vi "GEA2 Extract 2017 Washer.vi"(8 "Error In":errorcluster, 9 "ERD Number":u16 format="%x", 10 "Data":string, 11 "ERD Headers":string[](array[string])) -> (0 "Error Out":errorcluster, 3 "Array":string[][](array[string]))   [LabVIEW 2016, in "GEA2_Toolkit.lvlib"]
uses:
  library/GEA2_Toolkit.lvlib
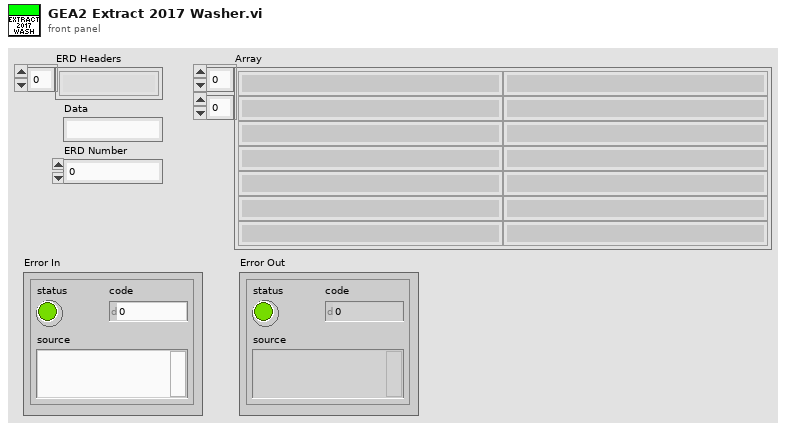
[diagram p1: front panel]
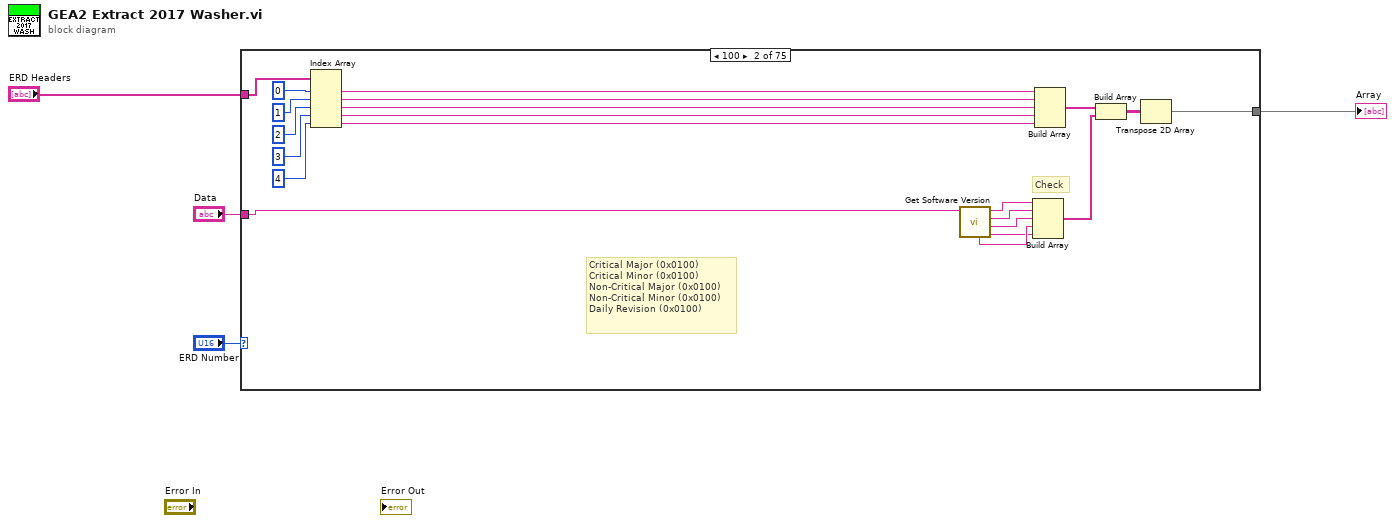
[diagram p0: block diagram]
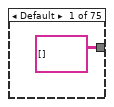
[diagram p2: hidden frame]
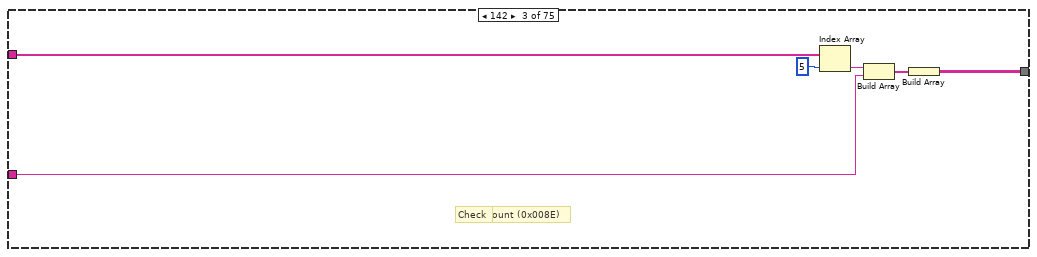
[diagram p3: hidden frame]
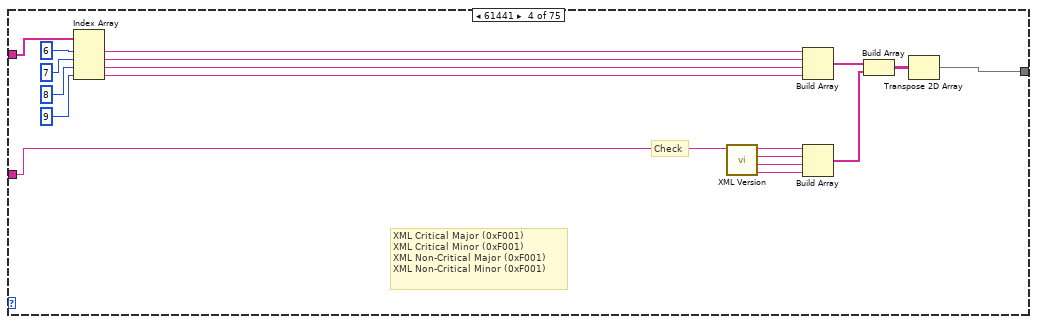
[diagram p4: hidden frame]
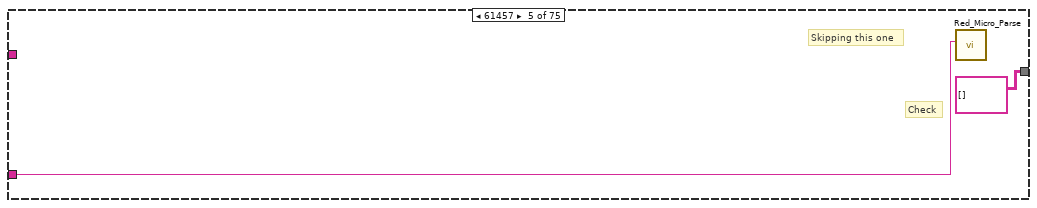
[diagram p5: hidden frame]
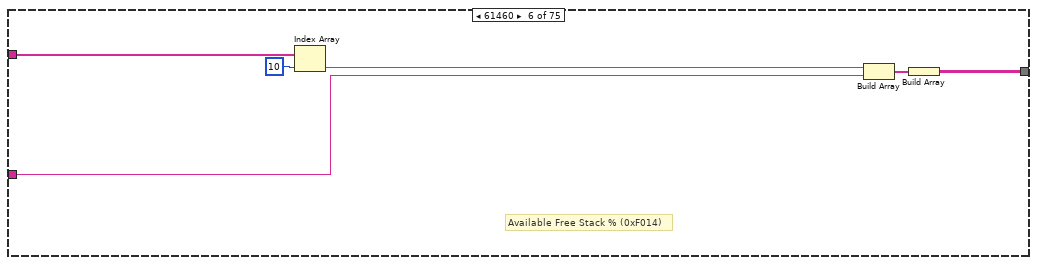
[diagram p6: hidden frame]
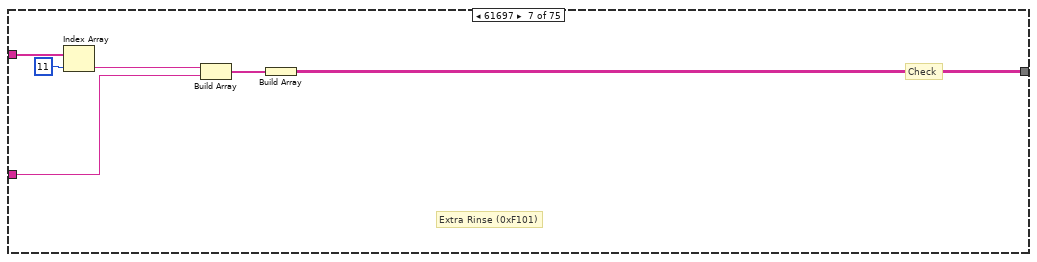
[diagram p7: hidden frame]
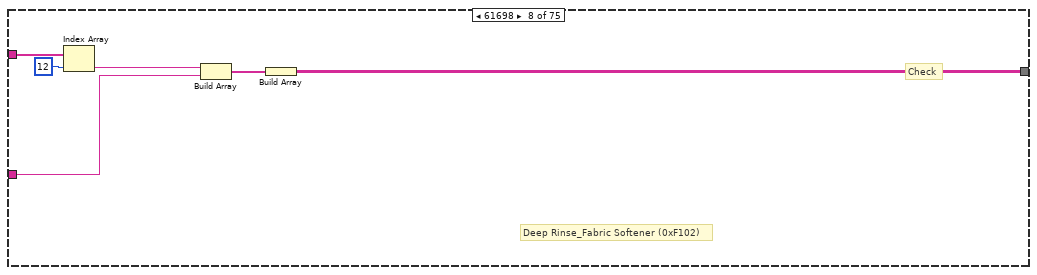
[diagram p8: hidden frame]
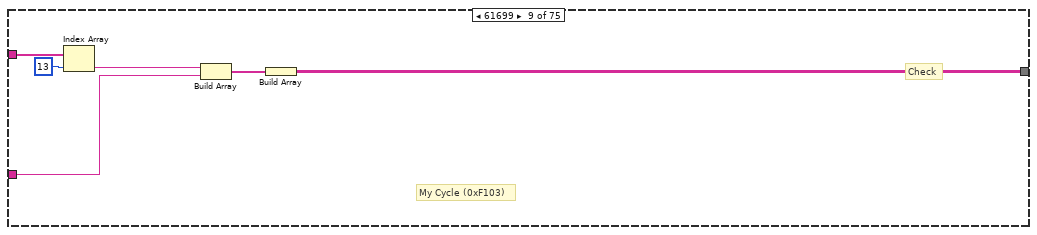
[diagram p9: hidden frame]
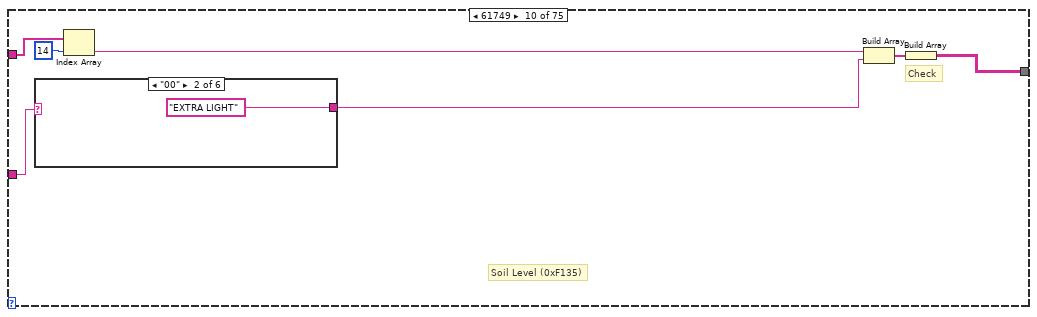
[diagram p10: hidden frame]
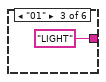
[diagram p12: hidden frame]
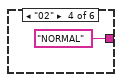
[diagram p13: hidden frame]
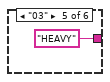
[diagram p14: hidden frame]
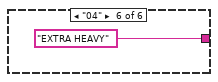
[diagram p15: hidden frame]
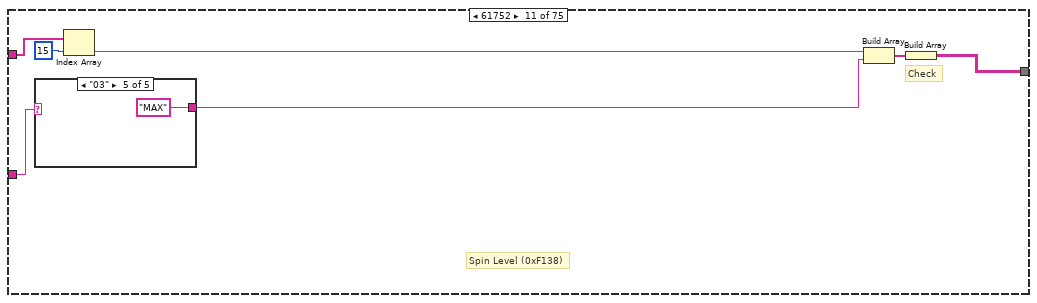
[diagram p16: hidden frame]
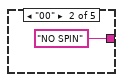
[diagram p18: hidden frame]
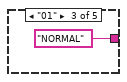
[diagram p19: hidden frame]
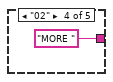
[diagram p20: hidden frame]
diagram:
  n1 = case shown="100" "ERD Number" {
    tunnel: "Data" -> [_ w26 w27 w50 w52 w53 w59 w65 w71 w83 w96 w108 w122 w136 w149 w157 w175 w181 w188 w199 w206 w212 w219 w230 w241 w252 w268 w282 w313 w323 w336 w342 w349 w364 w374 w384 w393 w409 w419 w424 w434 w444 w454 w464 w486 w500 w501 w508 w518 w527 w534 w540 w546 w553 w566 w588 w610 w625 w631 w638 w654 w671 w680 w686 w692 w709 w730 w737 w743 w749 w761 w762 w769 w775 w791]
    tunnel: [string[][] [] w6 w28 w33 string[][] [] w54 w60 w66 w72 w77 w90 w102 w116 w130 w143 w151 w176 w182 w187 w193 w207 w213 w224 w231 w242 w253 w262 w284 w288 w316 w330 w343 w350 w358 w368 w378 w394 w403 w413 w425 w435 w445 w455 w465 w473 w487 w503 w511 w519 w528 w535 w541 w547 w554 w559 w581 w603 w626 w632 w639 w647 w665 w681 w687 w693 w698 w724 w738 w744 w750 w756 w763 w770 w776 w781] -> w4
    tunnel: "ERD Headers" -> [_ w8 w32 w49 _ w58 w64 w67 w73 w79 w92 w103 w118 w132 w145 w153 w177 w183 w189 w195 w208 w214 w225 w232 w243 w255 w264 w285 w293 w319 w331 w344 w353 w359 w370 w380 w398 w404 w415 w428 w438 w446 w456 w468 w478 w492 w502 w512 w522 w530 w536 w542 w548 w555 w562 w582 w606 w627 w633 w640 w648 w667 w682 w688 w694 w701 w726 w739 w745 w751 w757 w764 w771 w777 w782]
    frame Default {
    }
    frame 256 {
      # "Critical Major (0x0100)\nCritical Minor (0x0100)\nNon-Critical Major (0x0100)\nNon-Critical Minor (0x0100)\nDaily Revision (0x0100)"
      # "Check"
      n2 = Index Array(array=w8, index #1=0 ("index"), index #2=1 ("index"), index #3=2 ("index"), index #4=3 ("index"), index #5=4 ("index")) -> (element #1=w20:string, element #2=w19:string, element #3=w18:string, element #4=w17:string, element #5=w16:string)
      n3 = call "Get Software Version.vi"("Data"=w26) -> ("Daily Revision"=w11:string, "Non-Critical Major"=w13:string, "Critical Minor"=w14:string, "Critical Major"=w15:string, "Non-Critical Minor"=w12:string)  [unwired: 6 in]
      n4 = Build Array(w15, w14, w13, w12, w11) -> (w9:string[])
      n5 = Build Array(w20, w19, w18, w17, w16) -> (w10:string[])
      n6 = Build Array(w10, w9) -> (w7:string[][])
      n7 = Transpose 2D Array(2D array=w7) -> (transposed array=w6:string[][])
    }
    frame 142 {
      # "Cycle Count (0x008E)"
      # "Check"
      n8 = Index Array(array=w32, index=5) -> (element=w30:string)
      n9 = Build Array(w30, w27) -> (w29:string[])
      n10 = Build Array(w29) -> (w28:string[][])
    }
    frame 61441 {
      # "XML Critical Major (0xF001)\nXML Critical Minor (0xF001)\nXML Non-Critical Major (0xF001)\nXML Non-Critical Minor (0xF001)"
      # "Check"
      n11 = Index Array(array=w49, index #1=6 ("index"), index #2=7 ("index"), index #3=8 ("index"), index #4=9 ("index")) -> (element #1=w44:string, element #2=w43:string, element #3=w42:string, element #4=w41:string)
      n12 = call "XML Version.vi"("Data"=w50) -> ("XML Non-Critical Minor"=w37:string, "XML Non-Critical Major"=w38:string, "XML Critical Minor"=w39:string, "XML Critical Major"=w40:string)  [unwired: 7 in]
      n13 = Build Array(w44, w43, w42, w41) -> (w36:string[])
      n14 = Build Array(w40, w39, w38, w37) -> (w35:string[])
      n15 = Build Array(w36, w35) -> (w34:string[][])
      n16 = Transpose 2D Array(2D array=w34) -> (transposed array=w33:string[][])
    }
    frame 61457 {
      # "Skipping this one"
      # "Check"
      n17 = call "Red_Micro_Parse.vi"("Data"=w52) -> ()  [unwired: 10 in, 1 out]
    }
    frame 61460 {
      # "Available Free Stack % (0xF014)"
      n18 = Index Array(array=w58, index=10) -> (element=w56:string)
      n19 = Build Array(w56, w53) -> (w55:string[])
      n20 = Build Array(w55) -> (w54:string[][])
    }
    frame 61697 {
      # "Extra Rinse (0xF101)"
      # "Check"
      n21 = Index Array(array=w64, index=11) -> (element=w62:string)
      n22 = Build Array(w62, w59) -> (w61:string[])
      n23 = Build Array(w61) -> (w60:string[][])
    }
    frame 61698 {
      # "Deep Rinse_Fabric Softener (0xF102)"
      # "Check"
      n24 = Index Array(array=w67, index=12) -> (element=w69:string)
      n25 = Build Array(w69, w65) -> (w68:string[])
      n26 = Build Array(w68) -> (w66:string[][])
    }
    frame 61699 {
      # "My Cycle (0xF103)"
      # "Check"
      n27 = Index Array(array=w73, index=13) -> (element=w75:string)
      n28 = Build Array(w75, w71) -> (w74:string[])
      n29 = Build Array(w74) -> (w72:string[][])
    }
    frame 61749 {
      # "Soil Level (0xF135)"
      # "Check"
      n30 = case shown="\"00\"" w83 {
        selector: w83 -> [w84 _ _ _ _ _]
        tunnel: [w84 "EXTRA LIGHT" "LIGHT" "NORMAL" "HEAVY" "EXTRA HEAVY"] -> w78
        frame Default {
        }
        frame "00" {
        }
        frame "01" {
        }
        frame "02" {
        }
        frame "03" {
        }
        frame "04" {
        }
      }
      n31 = Index Array(array=w79, index=14) -> (element=w81:string)
      n32 = Build Array(w81, w78) -> (w80:string[])
      n33 = Build Array(w80) -> (w77:string[][])
    }
    frame 61752 {
      # "Spin Level (0xF138)"
      # "Check"
      n34 = case shown="\"03\"" w96 {
        selector: w96 -> [w97 _ _ _ _]
        tunnel: [w97 "NO SPIN" "NORMAL" "MORE " "MAX"] -> w91
        frame Default {
        }
        frame "00" {
        }
        frame "01" {
        }
        frame "02" {
        }
        frame "03" {
        }
      }
      n35 = Index Array(array=w92, index=15) -> (element=w94:string)
      n36 = Build Array(w94, w91) -> (w93:string[])
      n37 = Build Array(w93) -> (w90:string[][])
    }
    frame 61751 {
      # "Stain (0xF137)"
      # "Check"
      n38 = case shown="Default" w108 {
        selector: w108 -> [w109 _ _ _ _ _ _]
        tunnel: [w109 "OFF" "TOMATO" "WINE" "BLOOD" "GRASS" "DIRT"] -> w104
        frame Default {
        }
        frame "00" {
        }
        frame "01" {
        }
        frame "02" {
        }
        frame "03" {
        }
        frame "04" {
        }
        frame "05" {
        }
      }
      n39 = Index Array(array=w103, index=16) -> (element=w106:string)
      n40 = Build Array(w106, w104) -> (w105:string[])
      n41 = Build Array(w105) -> (w102:string[][])
    }
    frame 61750 {
      # "Temperature Level (0xF136)"
      n42 = case shown="\"05\"" w122 {
        selector: w122 -> [w123 _ _ _ _ _ _]
        tunnel: [w123 "TAP COLD" "COLD" "COOL" "COLORS" "WARM" "HOT"] -> w117
        frame Default {
        }
        frame "00" {
        }
        frame "01" {
        }
        frame "02" {
        }
        frame "03" {
        }
        frame "04" {
        }
        frame "05" {
        }
      }
      n43 = Index Array(array=w118, index=17) -> (element=w120:string)
      n44 = Build Array(w120, w117) -> (w119:string[])
      n45 = Build Array(w119) -> (w116:string[][])
    }
    frame 61748 {
      # "Load Size (0xF134)"
      # "Check"
      n46 = case shown="\"04\"" w136 {
        selector: w136 -> [w137 _ _ _ _ _]
        tunnel: [w137 "SMALL" "MEDIUM" "LARGE" "SUPER" "PRECISE FILL"] -> w131
        frame Default {
        }
        frame "00" {
        }
        frame "01" {
        }
        frame "02" {
        }
        frame "03" {
        }
        frame "04" {
        }
      }
      n47 = Index Array(array=w132, index=18) -> (element=w134:string)
      n48 = Build Array(w134, w131) -> (w133:string[])
      n49 = Build Array(w133) -> (w130:string[][])
    }
    frame 61706 {
      # "Machine State (0xF10A)"
      # "Check"
      n50 = Decimal String To Number(string=w149) -> (number=w150:i32)  [unwired: 2 in, 1 out]
      n51 = Index Array(array=w145, index=19) -> (element=w147:string)
      n52 = call "Machine State.vi"("Numeric"=w150) -> ("Profile Status"=w144:string)  [unwired: 10 in]
      n53 = Build Array(w147, w144) -> (w146:string[])
      n54 = Build Array(w146) -> (w143:string[][])
    }
    frame 61708 {
      # "Cycle Selected (0xF10C)"
      # "Check"
      n55 = Decimal String To Number(string=w157) -> (number=w158:i32)  [unwired: 2 in, 1 out]
      n56 = Index Array(array=w153, index=20) -> (element=w155:string)
      n57 = case shown="3" w158 {
        tunnel: ["Cycle 0" ("Motor Profile") "Cycle 1" ("Motor Profile") "Cycle 2" ("Motor Profile") "Cycle 3" ("Motor Profile") "Cycle 4" ("Motor Profile") "Cycle 5" ("Motor Profile") "Cycle 6" ("Motor Profile") "Cycle 7" ("Motor Profile") "Cycle 8" ("Motor Profile") "Cycle 9" ("Motor Profile") "Cycle 10" ("Motor Profile") "Cycle 11" ("Motor Profile") "Cycle 12" ("Motor Profile") "Cycle 13" ("Motor Profile") "Cycle 14" ("Motor Profile") "Cycle 15" ("Motor Profile")] -> w152
        frame 0, Default {
        }
        frame 1 {
        }
        frame 2 {
        }
        frame 3 {
        }
        frame 4 {
        }
        frame 5 {
        }
        frame 6 {
        }
        frame 7 {
        }
        frame 8 {
        }
        frame 9 {
        }
        frame 10 {
        }
        frame 11 {
        }
        frame 12 {
        }
        frame 13 {
        }
        frame 14 {
        }
        frame 15 {
        }
      }
      n58 = Build Array(w155, w152) -> (w154:string[])
      n59 = Build Array(w154) -> (w151:string[][])
    }
    frame 61709 {
      # "Delay Time (0xF10D)"
      # "Might not work"
      n60 = Index Array(array=w177, index=21) -> (element=w179:string)
      n61 = Build Array(w179, w175) -> (w178:string[])
      n62 = Build Array(w178) -> (w176:string[][])
    }
    frame 61710 {
      # "Soak Time (0xF10E)"
      # "Check"
      n63 = Index Array(array=w183, index=22) -> (element=w185:string)
      n64 = Build Array(w185, w181) -> (w184:string[])
      n65 = Build Array(w184) -> (w182:string[][])
    }
    frame 61726 {
      # "Auto Soak Level (0xF11E)"
      # "Check"
      n66 = Index Array(array=w189, index=23) -> (element=w191:string)
      n67 = Build Array(w191, w188) -> (w190:string[])
      n68 = Build Array(w190) -> (w187:string[][])
    }
    frame 61731 {
      # "Deep Fill (0xF123)"
      # "Check. Could add names:\n00=Off\n01=Incremental Fill\n02=Max Fill"
      n69 = Index Array(array=w195, index=24) -> (element=w197:string)
      n70 = case shown="\"02\"" w199 {
        tunnel: [FALSE ("Eco Wash") TRUE ("Eco Wash") TRUE ("Eco Wash")] -> _
        tunnel: ["Off" "Incremental Fill" "Max Fill"] -> w194
        frame "00", Default {
        }
        frame "01" {
        }
        frame "02" {
        }
      }
      n71 = Build Array(w197, w194) -> (w196:string[])
      n72 = Build Array(w196) -> (w193:string[][])
    }
    frame 61732 {
      # "Warm Rinse (0xF124)"
      # "Check"
      n73 = Index Array(array=w208, index=25) -> (element=w210:string)
      n74 = Build Array(w210, w206) -> (w209:string[])
      n75 = Build Array(w209) -> (w207:string[][])
    }
    frame 61760 {
      # "Remaining Cycle Time(s) (0xF140)"
      # "Check"
      n76 = Index Array(array=w214, index=26) -> (element=w216:string)
      n77 = Build Array(w216, w212) -> (w215:string[])
      n78 = Build Array(w215) -> (w213:string[][])
    }
    frame 61952 {
      # "Wet Load Gallons (0xF200)"
      # "Check"
      n79 = Index Array(array=w225, index=27) -> (element=w227:string)
      n80 = Fract/Exp String To Number(string=w219) -> (number=w218:dbl)  [unwired: 3 in, 1 out]
      n81 = Divide(x=w218, y=100.0) -> (x/y=w223:dbl)
      n82 = Number To Fractional String(number=w223, precision (6)=i16 3) -> (F-format string=w220:string)  [unwired: 2 in]
      n83 = Build Array(w227, w220) -> (w226:string[])
      n84 = Build Array(w226) -> (w224:string[][])
    }
    frame 61953 {
      # "Tub Volume Gallons (0xF201)"
      # "Check"
      n85 = Index Array(array=w232, index=28) -> (element=w237:string)
      n86 = Fract/Exp String To Number(string=w230) -> (number=w229:dbl)  [unwired: 3 in, 1 out]
      n87 = Divide(x=w229, y=100.0) -> (x/y=w233:dbl)
      n88 = Number To Fractional String(number=w233, precision (6)=i16 3) -> (F-format string=w234:string)  [unwired: 2 in]
      n89 = Build Array(w237, w234) -> (w236:string[])
      n90 = Build Array(w236) -> (w231:string[][])
    }
    frame 61954 {
      # "Pressure (inches of H20) (0xF202)"
      n91 = Index Array(array=w243, index=29) -> (element=w248:string)
      n92 = Fract/Exp String To Number(string=w241) -> (number=w240:dbl)  [unwired: 3 in, 1 out]
      n93 = Divide(x=w240, y=1000.0) -> (x/y=w244:dbl)
      n94 = Number To Fractional String(number=w244, precision (6)=i16 3) -> (F-format string=w245:string)  [unwired: 2 in]
      n95 = Build Array(w248, w245) -> (w247:string[])
      n96 = Build Array(w247) -> (w242:string[][])
    }
    frame 61957 {
      # "Target Gallons (0xF205)"
      # "Check"
      n97 = Index Array(array=w255, index=30) -> (element=w259:string)
      n98 = Fract/Exp String To Number(string=w252) -> (number=w251:dbl)  [unwired: 3 in, 1 out]
      n99 = Divide(x=w251, y=100.0) -> (x/y=w254:dbl)
      n100 = Number To Fractional String(number=w254, precision (6)=i16 3) -> (F-format string=w256:string)  [unwired: 2 in]
      n101 = Build Array(w259, w256) -> (w258:string[])
      n102 = Build Array(w258) -> (w253:string[][])
    }
    frame 61958 {
      # "Load Type (0xF206)"
      # "Check....could use the U8 conversion"
      n103 = case shown="\"0\"" w268 {
        selector: w268 -> [w269 _ _ _ _ _ _ _ _ _ _ _ _]
        tunnel: [w269 "UNKNOWN" "COTTON" "SYNTHETIC" "MIXED" "WET" "LOW FLOW" "SMALL" "MEDIUM" "LARGE" "SUPER" "SUPER PLUS" "MAX"] -> w263
        frame Default {
        }
        frame "0" {
        }
        frame "1" {
        }
        frame "2" {
        }
        frame "3" {
        }
        frame "4" {
        }
        frame "5" {
        }
        frame "6" {
        }
        frame "7" {
        }
        frame "8" {
        }
        frame "9" {
        }
        frame "10" {
        }
        frame "11" {
        }
      }
      n104 = Index Array(array=w264, index=31) -> (element=w266:string)
      n105 = Build Array(w266, w263) -> (w265:string[])
      n106 = Build Array(w265) -> (w262:string[][])
    }
    frame 61959 {
      # "Lid Switch (0xF207)"
      # "Check"
      n107 = Index Array(array=w285, index=32) -> (element=w287:string)
      n108 = Build Array(w287, w282) -> (w286:string[])
      n109 = Build Array(w286) -> (w284:string[][])
    }
    frame 61961 {
      # "Hot Water Valve (0xF209)\nCold Water Valve (0xF209)\nSpray_Rinse Valve (0xF209)\nFabric Softener Valve (0xF209)"
      # "Check"
      n110 = Index Array(array=w293, index #1=33 ("index"), index #2=34 ("index"), index #3=35 ("index"), index #4=36 ("index")) -> (element #1=w300:string, element #2=w299:string, element #3=w298:string, element #4=w297:string)
      n111 = Decimal String To Number(string=w313) -> (number=w314:i32)  [unwired: 2 in, 1 out]
      n112 = Number To Boolean Array(number=w314) -> (Boolean array=w315:bool[])
      n113 = Index Array(array=w315) -> (element #1=w308:bool, element #2=w307:bool, element #3=w306:bool, element #4=w305:bool)  [unwired: 4 in]
      n114 = Boolean To (0,1)(Boolean=w308) -> (0, 1=w312:i16)
      n115 = Boolean To (0,1)(Boolean=w307) -> (0, 1=w311:i16)
      n116 = Boolean To (0,1)(Boolean=w306) -> (0, 1=w310:i16)
      n117 = Boolean To (0,1)(Boolean=w305) -> (0, 1=w309:i16)
      n118 = Number To Decimal String(number=w312) -> (decimal integer string=w292:string)  [unwired: 1 in]
      n119 = Number To Decimal String(number=w311) -> (decimal integer string=w291:string)  [unwired: 1 in]
      n120 = Number To Decimal String(number=w310) -> (decimal integer string=w290:string)  [unwired: 1 in]
      n121 = Number To Decimal String(number=w309) -> (decimal integer string=w289:string)  [unwired: 1 in]
      n122 = Build Array(w300, w299, w298, w297) -> (w296:string[])
      n123 = Build Array(w292, w291, w290, w289) -> (w295:string[])
      n124 = Build Array(w296, w295) -> (w294:string[][])
      n125 = Transpose 2D Array(2D array=w294) -> (transposed array=w288:string[][])
    }
    frame 61962 {
      # "Lid Lock Req State (0xF20A)"
      # "Check"
      n126 = String Subset(string=w323, offset (0)=3, length (rest)=2 ("length (rest)")) -> (substring=w324:string)
      n127 = Index Array(array=w319, index=37) -> (element=w321:string)
      n128 = Hexadecimal String To Number(string=w324) -> (number=w322:u32)  [unwired: 2 in, 1 out]
      n129 = case shown="2" w322 {
        tunnel: ["UNLOCKED" "LOCKED" "FAILURE"] -> w317
        frame 0, Default {
        }
        frame 1 {
        }
        frame 2 {
        }
      }
      n130 = Build Array(w321, w317) -> (w320:string[])
      n131 = Build Array(w320) -> (w316:string[][])
    }
    frame 61963 {
      # "Lid Lock Status (0xF20B)"
      # "Check"
      n132 = Decimal String To Number(string=w336) -> (number=w337:i32)  [unwired: 2 in, 1 out]
      n133 = Index Array(array=w331, index=38) -> (element=w334:string)
      n134 = case shown="2" w337 {
        tunnel: ["Unlocked" ("Motor Profile") "Locked" ("Motor Profile") "Failure" ("Motor Profile")] -> w332
        frame 0, Default {
        }
        frame 1 {
        }
        frame 2 {
        }
      }
      n135 = Build Array(w334, w332) -> (w333:string[])
      n136 = Build Array(w333) -> (w330:string[][])
    }
    frame 61964 {
      # "Cycle Engine State (0xF20C)"
      n137 = Index Array(array=w344, index=39) -> (element=w346:string)
      n138 = call "Cycle Engine State.vi"("Data"=w342) -> ("Cycle Engine State"=w341:string)  [unwired: 10 in]
      n139 = Build Array(w346, w341) -> (w345:string[])
      n140 = Build Array(w345) -> (w343:string[][])
    }
    frame 61967 {
      # "Current Water Temperature (°F) (0xF20F)"
      # "Check"
      n141 = Index Array(array=w353, index=40) -> (element=w355:string)
      n142 = Fract/Exp String To Number(string=w349) -> (number=w348:dbl)  [unwired: 3 in, 1 out]
      n143 = Divide(x=w348, y=10.0) -> (x/y=w352:dbl)
      n144 = Number To Fractional String(number=w352) -> (F-format string=w351:string)  [unwired: 3 in]
      n145 = Build Array(w355, w351) -> (w354:string[])
      n146 = Build Array(w354) -> (w350:string[][])
    }
    frame 61968 {
      # "Drain Pump (0xF210)"
      # "Check"
      n147 = String Subset(string=w364, offset (0)=3, length (rest)=2 ("length (rest)")) -> (substring=w365:string)
      n148 = Index Array(array=w359, index=41) -> (element=w362:string)
      n149 = call "HexStringToBoolean.vi"("Hex String"=w365) -> ("decimal integer string"=w360:string)  [unwired: 1 in, 1 out]
      n150 = Build Array(w362, w360) -> (w361:string[])
      n151 = Build Array(w361) -> (w358:string[][])
    }
    frame 61969 {
      # "Recirculating Pump (0xF211)"
      n152 = String Subset(string=w374, offset (0)=3, length (rest)=2 ("length (rest)")) -> (substring=w375:string)
      n153 = Index Array(array=w370, index=42) -> (element=w372:string)
      n154 = call "HexStringToBoolean.vi"("Hex String"=w375) -> ("decimal integer string"=w369:string)  [unwired: 1 in, 1 out]
      n155 = Build Array(w372, w369) -> (w371:string[])
      n156 = Build Array(w371) -> (w368:string[][])
    }
    frame 61971 {
      # "Sub-Cycle (0xF213)"
      # "Check"
      n157 = case shown="\"04\"" w384 {
        selector: w384 -> [w385 _ _ _ _ _ _]
        tunnel: [w385 "NONE" "FILL" "SOAK" "WASH" "RINSE" "SPIN"] -> w379
        frame Default {
        }
        frame "00" {
        }
        frame "01" {
        }
        frame "02" {
        }
        frame "04" {
        }
        frame "08" {
        }
        frame "10" {
        }
      }
      n158 = Index Array(array=w380, index=43) -> (element=w382:string)
      n159 = Build Array(w382, w379) -> (w381:string[])
      n160 = Build Array(w381) -> (w378:string[][])
    }
    frame 61973 {
      # "Target Level Inches (0xF215)"
      # "Check"
      n161 = Index Array(array=w398, index=44) -> (element=w400:string)
      n162 = Fract/Exp String To Number(string=w393) -> (number=w392:dbl)  [unwired: 3 in, 1 out]
      n163 = Divide(x=w392, y=1000.0) -> (x/y=w397:dbl)
      n164 = Number To Fractional String(number=w397, precision (6)=i16 3) -> (F-format string=w395:string)  [unwired: 2 in]
      n165 = Build Array(w400, w395) -> (w399:string[])
      n166 = Build Array(w399) -> (w394:string[][])
    }
    frame 61976 {
      # "Valve Relay (0xF218)"
      # "Check"
      n167 = String Subset(string=w409, offset (0)=3, length (rest)=2 ("length (rest)")) -> (substring=w410:string)
      n168 = Index Array(array=w404, index=45) -> (element=w407:string)
      n169 = call "HexStringToBoolean.vi"("Hex String"=w410) -> ("decimal integer string"=w405:string)  [unwired: 1 in, 1 out]
      n170 = Build Array(w407, w405) -> (w406:string[])
      n171 = Build Array(w406) -> (w403:string[][])
    }
    frame 61977 {
      # "Lid Lock FB (0xF219)"
      # "Check"
      n172 = case shown="\"01\"" w419 {
        selector: w419 -> [w420 _ _]
        tunnel: [w420 "LOCKED" ("Motor Profile") "UNLOCKED" ("Motor Profile")] -> w414
        frame "0", Default {
        }
        frame "00" {
        }
        frame "01" {
        }
      }
      n173 = Index Array(array=w415, index=46) -> (element=w417:string)
      n174 = Build Array(w417, w414) -> (w416:string[])
      n175 = Build Array(w416) -> (w413:string[][])
    }
    frame 61985 {
      # "Target Bath Temperature (°F) (0xF221)"
      # "Check"
      n176 = Index Array(array=w428, index=47) -> (element=w430:string)
      n177 = Fract/Exp String To Number(string=w424) -> (number=w423:dbl)  [unwired: 3 in, 1 out]
      n178 = Divide(x=w423, y=10.0) -> (x/y=w427:dbl)
      n179 = Number To Fractional String(number=w427) -> (F-format string=w426:string)  [unwired: 3 in]
      n180 = Build Array(w430, w426) -> (w429:string[])
      n181 = Build Array(w429) -> (w425:string[][])
    }
    frame 61986 {
      # "Current Bath Temperature (°F) (0xF222)"
      # "Check"
      n182 = Index Array(array=w438, index=48) -> (element=w440:string)
      n183 = Fract/Exp String To Number(string=w434) -> (number=w433:dbl)  [unwired: 3 in, 1 out]
      n184 = Divide(x=w433, y=10.0) -> (x/y=w437:dbl)
      n185 = Number To Fractional String(number=w437) -> (F-format string=w436:string)  [unwired: 3 in]
      n186 = Build Array(w440, w436) -> (w439:string[])
      n187 = Build Array(w439) -> (w435:string[][])
    }
    frame 61987 {
      # "Cold Inlet Temperature (°F) (0xF223)"
      # "Check"
      n188 = Index Array(array=w446, index=49) -> (element=w450:string)
      n189 = Fract/Exp String To Number(string=w444) -> (number=w443:dbl)  [unwired: 3 in, 1 out]
      n190 = Divide(x=w443, y=10.0) -> (x/y=w448:dbl)
      n191 = Number To Fractional String(number=w448) -> (F-format string=w447:string)  [unwired: 3 in]
      n192 = Build Array(w450, w447) -> (w449:string[])
      n193 = Build Array(w449) -> (w445:string[][])
    }
    frame 61988 {
      # "Hot Inlet Temperature (°F) (0xF224)"
      # "Check"
      n194 = Index Array(array=w456, index=50) -> (element=w460:string)
      n195 = Fract/Exp String To Number(string=w454) -> (number=w453:dbl)  [unwired: 3 in, 1 out]
      n196 = Divide(x=w453, y=10.0) -> (x/y=w458:dbl)
      n197 = Number To Fractional String(number=w458) -> (F-format string=w457:string)  [unwired: 3 in]
      n198 = Build Array(w460, w457) -> (w459:string[])
      n199 = Build Array(w459) -> (w455:string[][])
    }
    frame 61989 {
      # "Warm Inlet Temperature (°F) (0xF225)"
      # "Check"
      n200 = Index Array(array=w468, index=51) -> (element=w470:string)
      n201 = Fract/Exp String To Number(string=w464) -> (number=w463:dbl)  [unwired: 3 in, 1 out]
      n202 = Divide(x=w463, y=10.0) -> (x/y=w467:dbl)
      n203 = Number To Fractional String(number=w467) -> (F-format string=w466:string)  [unwired: 3 in]
      n204 = Build Array(w470, w466) -> (w469:string[])
      n205 = Build Array(w469) -> (w465:string[][])
    }
    frame 61990 {
      # "Hot Gallons (0xF226)\nCold Gallons (0xF226)"
      # "Check"
      # "Check"
      n206 = call "Hot and Cold Gallons.vi"("Data"=w486) -> ("ColdGallons"=w476:dbl, "Hot Gallons"=w477:dbl)  [unwired: 9 in]
      n207 = Index Array(array=w478, index #1=52 ("index"), index #2=53 ("index")) -> (element #1=w483:string, element #2=w482:string)
      n208 = Number To Fractional String(number=w477) -> (F-format string=w475:string)  [unwired: 3 in]
      n209 = Number To Fractional String(number=w476) -> (F-format string=w474:string)  [unwired: 3 in]
      n210 = Build Array(w483, w482) -> (w481:string[])
      n211 = Build Array(w475, w474) -> (w480:string[])
      n212 = Build Array(w481, w480) -> (w479:string[][])
      n213 = Transpose 2D Array(2D array=w479) -> (transposed array=w473:string[][])
    }
    frame 61991 {
      # "Hot Seg Valve Time (0xF227)\nCold Seg Valve Time (0xF227)"
      # "Check"
      # "Check"
      n214 = Index Array(array=w492, index #1=54 ("index"), index #2=55 ("index")) -> (element #1=w497:string, element #2=w496:string)
      n215 = call "Segment Valve Time.vi"("Data"=w500) -> ("Cold Segment Valve Time"=w488:u16, "Hot Segment Valve Time"=w489:u16)  [unwired: 9 in]
      n216 = Number To Decimal String(number=w489) -> (decimal integer string=w491:string)  [unwired: 1 in]
      n217 = Number To Decimal String(number=w488) -> (decimal integer string=w490:string)  [unwired: 1 in]
      n218 = Build Array(w491, w490) -> (w494:string[])
      n219 = Build Array(w497, w496) -> (w495:string[])
      n220 = Build Array(w495, w494) -> (w493:string[][])
      n221 = Transpose 2D Array(2D array=w493) -> (transposed array=w487:string[][])
    }
    frame 61994 {
      # "Child Safety (0xF22A)"
      # "Check"
      n222 = Index Array(array=w502, index=56) -> (element=w505:string)
      n223 = Build Array(w505, w501) -> (w504:string[])
      n224 = Build Array(w504) -> (w503:string[][])
    }
    frame 61995 {
      # "Segment Gallons (0xF22B)"
      # "Check"
      n225 = Index Array(array=w512, index=57) -> (element=w514:string)
      n226 = Fract/Exp String To Number(string=w508) -> (number=w507:dbl)  [unwired: 3 in, 1 out]
      n227 = Divide(x=w507, y=100.0) -> (x/y=w510:dbl)
      n228 = Number To Fractional String(number=w510) -> (F-format string=w509:string)  [unwired: 3 in]
      n229 = Build Array(w514, w509) -> (w513:string[])
      n230 = Build Array(w513) -> (w511:string[][])
    }
    frame 62208 {
      # "Ramp Average Current (0xF300)"
      # "Check"
      n231 = Fract/Exp String To Number(string=w518) -> (number=w517:dbl)  [unwired: 3 in, 1 out]
      n232 = Index Array(array=w522, index=58) -> (element=w524:string)
      n233 = Divide(x=w517, y=1024.0) -> (x/y=w521:dbl)
      n234 = Number To Fractional String(number=w521) -> (F-format string=w520:string)  [unwired: 3 in]
      n235 = Build Array(w524, w520) -> (w523:string[])
      n236 = Build Array(w523) -> (w519:string[][])
    }
    frame 62209 {
      # "Coast Line Voltage (0xF301)"
      # "Check"
      n237 = Index Array(array=w530, index=59) -> (element=w532:string)
      n238 = call "Q5 Format.vi"("Data (U16 or U32)"=w527) -> ("Q5 Format Data"=w529:string)  [unwired: 10 in]
      n239 = Build Array(w532, w529) -> (w531:string[])
      n240 = Build Array(w531) -> (w528:string[][])
    }
    frame 62210 {
      # "Ramp Speed (0xF302)"
      # "Check"
      n241 = Index Array(array=w536, index=60) -> (element=w538:string)
      n242 = Build Array(w538, w534) -> (w537:string[])
      n243 = Build Array(w537) -> (w535:string[][])
    }
    frame 62211 {
      # "Ramp Time (0xF303)"
      # "Check"
      n244 = Index Array(array=w542, index=61) -> (element=w544:string)
      n245 = Build Array(w544, w540) -> (w543:string[])
      n246 = Build Array(w543) -> (w541:string[][])
    }
    frame 62212 {
      # "Coast Time (0xF304)"
      # "Check"
      n247 = Index Array(array=w548, index=62) -> (element=w550:string)
      n248 = Build Array(w550, w546) -> (w549:string[])
      n249 = Build Array(w549) -> (w547:string[][])
    }
    frame 62213 {
      # "Dry Load Size (0xF305)"
      # "Check"
      n250 = Index Array(array=w555, index=63) -> (element=w557:string)
      n251 = call "Q5 Format.vi"("Data (U16 or U32)"=w553) -> ("Q5 Format Data"=w552:string)  [unwired: 10 in]
      n252 = Build Array(w557, w552) -> (w556:string[])
      n253 = Build Array(w556) -> (w554:string[][])
    }
    frame 62214 {
      # "Folding in Acceleration (0xF306)"
      # "Check"
      n254 = String Subset(string=w566, offset (0)=0, length (rest)=2 ("length (rest)")) -> (substring=w576:string)
      n255 = String Subset(string=w566, offset (0)=3, length (rest)=2 ("length (rest)")) -> (substring=w575:string)
      n256 = String Subset(string=w566, offset (0)=6, length (rest)=2 ("length (rest)")) -> (substring=w568:string)
      n257 = String Subset(string=w566, offset (0)=9, length (rest)=2 ("length (rest)")) -> (substring=w567:string)
      n258 = Index Array(array=w562, index=64) -> (element=w564:string)
      n259 = Concatenate Strings(w576, w575, w568, w567) -> (w574:string)
      n260 = Hexadecimal String To Number(string=w574) -> (number=w573:u32)  [unwired: 2 in, 1 out]
      n261 = To Long Integer(number=w573) -> (32bit integer=w561:i32)
      n262 = Number To Decimal String(number=w561) -> (decimal integer string=w560:string)  [unwired: 1 in]
      n263 = Build Array(w564, w560) -> (w563:string[])
      n264 = Build Array(w563) -> (w559:string[][])
    }
    frame 62215 {
      # "Max Jerk In Acceleration (0xF307)"
      # "Check"
      n265 = String Subset(string=w588, offset (0)=0, length (rest)=2 ("length (rest)")) -> (substring=w598:string)
      n266 = String Subset(string=w588, offset (0)=3, length (rest)=2 ("length (rest)")) -> (substring=w597:string)
      n267 = String Subset(string=w588, offset (0)=6, length (rest)=2 ("length (rest)")) -> (substring=w590:string)
      n268 = String Subset(string=w588, offset (0)=9, length (rest)=2 ("length (rest)")) -> (substring=w589:string)
      n269 = Index Array(array=w582, index=65) -> (element=w586:string)
      n270 = Concatenate Strings(w598, w597, w590, w589) -> (w596:string)
      n271 = Hexadecimal String To Number(string=w596) -> (number=w595:u32)  [unwired: 2 in, 1 out]
      n272 = To Long Integer(number=w595) -> (32bit integer=w584:i32)
      n273 = Number To Decimal String(number=w584) -> (decimal integer string=w583:string)  [unwired: 1 in]
      n274 = Build Array(w586, w583) -> (w585:string[])
      n275 = Build Array(w585) -> (w581:string[][])
    }
    frame 62216 {
      # "Max Jerk In S-S (0xF308)"
      # "Check"
      n276 = String Subset(string=w610, offset (0)=0, length (rest)=2 ("length (rest)")) -> (substring=w620:string)
      n277 = String Subset(string=w610, offset (0)=3, length (rest)=2 ("length (rest)")) -> (substring=w619:string)
      n278 = String Subset(string=w610, offset (0)=6, length (rest)=2 ("length (rest)")) -> (substring=w612:string)
      n279 = String Subset(string=w610, offset (0)=9, length (rest)=2 ("length (rest)")) -> (substring=w611:string)
      n280 = Index Array(array=w606, index=66) -> (element=w608:string)
      n281 = Concatenate Strings(w620, w619, w612, w611) -> (w618:string)
      n282 = Hexadecimal String To Number(string=w618) -> (number=w617:u32)  [unwired: 2 in, 1 out]
      n283 = To Long Integer(number=w617) -> (32bit integer=w605:i32)
      n284 = Number To Decimal String(number=w605) -> (decimal integer string=w604:string)  [unwired: 1 in]
      n285 = Build Array(w608, w604) -> (w607:string[])
      n286 = Build Array(w607) -> (w603:string[][])
    }
    frame 62218 {
      # "Shaft Speed (RPM) (0xF30A)"
      n287 = Index Array(array=w627, index=67) -> (element=w629:string)
      n288 = Build Array(w629, w625) -> (w628:string[])
      n289 = Build Array(w628) -> (w626:string[][])
    }
    frame 62219 {
      # "Basket Speed (RPM) (0xF30B)"
      # "Check"
      n290 = Index Array(array=w633, index=68) -> (element=w635:string)
      n291 = Build Array(w635, w631) -> (w634:string[])
      n292 = Build Array(w634) -> (w632:string[][])
    }
    frame 62221 {
      # "Current RMS (Amps) (0xF30D)"
      n293 = Fract/Exp String To Number(string=w638) -> (number=w637:dbl)  [unwired: 3 in, 1 out]
      n294 = Divide(x=w637, y=1024.0) -> (x/y=w642:dbl)
      n295 = Index Array(array=w640, index=69) -> (element=w644:string)
      n296 = Number To Fractional String(number=w642) -> (F-format string=w641:string)  [unwired: 3 in]
      n297 = Build Array(w644, w641) -> (w643:string[])
      n298 = Build Array(w643) -> (w639:string[][])
    }
    frame 62222 {
      # "Target Speed (RPM) (0xF30E)"
      # "Check"
      n299 = String Subset(string=w654, offset (0)=0, length (rest)=2 ("length (rest)")) -> (substring=w660:string)
      n300 = String Subset(string=w654, offset (0)=3, length (rest)=2 ("length (rest)")) -> (substring=w659:string)
      n301 = Concatenate Strings(w660, w659) -> (w658:string)
      n302 = Hexadecimal String To Number(string=w658) -> (number=w657:u32)  [unwired: 2 in, 1 out]
      n303 = To Word Integer(number=w657) -> (16bit integer=w656:i16)
      n304 = Absolute Value(x=w656) -> (abs(x)=w655:i16)
      n305 = To Unsigned Word Integer(number=w655) -> (unsigned 16bit integer=w650:u16)
      n306 = Index Array(array=w648, index=70) -> (element=w652:string)
      n307 = Number To Decimal String(number=w650) -> (decimal integer string=w649:string)  [unwired: 1 in]
      n308 = Build Array(w652, w649) -> (w651:string[])
      n309 = Build Array(w651) -> (w647:string[][])
    }
    frame 62227 {
      # "Motor Mode (0xF313)"
      # "Check"
      n310 = Decimal String To Number(string=w671) -> (number=w672:i32)  [unwired: 2 in, 1 out]
      n311 = Index Array(array=w667, index=71) -> (element=w669:string)
      n312 = case shown="3" w672 {
        tunnel: ["Closed Loop" "Closed Loop Angle" "Open Loop" "Open Loop Angle" "Coasting" "Braking" "Idle"] -> w666
        frame 0, Default {
        }
        frame 1 {
        }
        frame 2 {
        }
        frame 3 {
        }
        frame 4 {
        }
        frame 5 {
        }
        frame 6 {
        }
      }
      n313 = Build Array(w669, w666) -> (w668:string[])
      n314 = Build Array(w668) -> (w665:string[][])
    }
    frame 62229 {
      # "OOB Detected in Acceleration (0xF315)"
      # "Check"
      n315 = Index Array(array=w682, index=72) -> (element=w684:string)
      n316 = Build Array(w684, w680) -> (w683:string[])
      n317 = Build Array(w683) -> (w681:string[][])
    }
    frame 62230 {
      # "OOB Detected in S-S (0xF316)"
      # "Check"
      n318 = Index Array(array=w688, index=73) -> (element=w690:string)
      n319 = Build Array(w690, w686) -> (w689:string[])
      n320 = Build Array(w689) -> (w687:string[][])
    }
    frame 62231 {
      # "OOB ReDistribution Required (0xF317)"
      # "Check"
      n321 = Index Array(array=w694, index=74) -> (element=w696:string)
      n322 = Build Array(w696, w692) -> (w695:string[])
      n323 = Build Array(w695) -> (w693:string[][])
    }
    frame 62233 {
      # "Motor Profile Status (0xF319)\nMotor Profile (0xF319)"
      # "Check"
      # "Check"
      n324 = String Subset(string=w709, offset (0)=3, length (rest)=2 ("length (rest)")) -> (substring=w714:string)
      n325 = String Subset(string=w709, offset (0)=0, length (rest)=2 ("length (rest)")) -> (substring=w711:string)
      n326 = Index Array(array=w701, index #1=75 ("index"), index #2=76 ("index")) -> (element #1=w706:string, element #2=w705:string)
      n327 = case shown="\"06\"" w714 {
        tunnel: ["Unknown" ("Profile Status") "Started" ("Profile Status") "Stopped" ("Profile Status") "Paused" ("Profile Status") "Resumed" ("Profile Status") "Selected" ("Profile Status") "Completed" ("Profile Status")] -> w700
        frame "00", Default {
        }
        frame "06" {
        }
        frame "07" {
        }
        frame "08" {
        }
        frame "09" {
        }
        frame "0A" {
        }
        frame "0B" {
        }
      }
      n328 = Hexadecimal String To Number(string=w711) -> (number=w710:u32)  [unwired: 2 in, 1 out]
      n329 = Number To Decimal String(number=w710) -> (decimal integer string=w699:string)  [unwired: 1 in]
      n330 = Build Array(w706, w705) -> (w704:string[])
      n331 = Build Array(w700, w699) -> (w703:string[])
      n332 = Build Array(w704, w703) -> (w702:string[][])
      n333 = Transpose 2D Array(2D array=w702) -> (transposed array=w698:string[][])
    }
    frame 62237 {
      # "Mode Shift Status (0xF31D)"
      # "Check"
      n334 = Decimal String To Number(string=w730) -> (number=w731:i32)  [unwired: 2 in, 1 out]
      n335 = Index Array(array=w726, index=77) -> (element=w728:string)
      n336 = case shown="1" w731 {
        tunnel: ["Unknown" ("Motor Profile") "Agitate State" ("Motor Profile") "Spin State" ("Motor Profile") "Trans to Spin" ("Motor Profile") "Trans to Agitate" ("Motor Profile")] -> w725
        frame 0, Default {
        }
        frame 1 {
        }
        frame 2 {
        }
        frame 3 {
        }
        frame 4 {
        }
      }
      n337 = Build Array(w728, w725) -> (w727:string[])
      n338 = Build Array(w727) -> (w724:string[][])
    }
    frame 62241 {
      # "ME Relay (0xF321)"
      # "Check"
      n339 = Index Array(array=w739, index=78) -> (element=w741:string)
      n340 = Build Array(w741, w737) -> (w740:string[])
      n341 = Build Array(w740) -> (w738:string[][])
    }
    frame 62242 {
      # "Mode Shift FB (0xF322)"
      # "Check"
      n342 = Index Array(array=w745, index=79) -> (element=w747:string)
      n343 = Build Array(w747, w743) -> (w746:string[])
      n344 = Build Array(w746) -> (w744:string[][])
    }
    frame 62243 {
      # "MS Motor (0xF323)"
      # "Check"
      n345 = Index Array(array=w751, index=80) -> (element=w753:string)
      n346 = Build Array(w753, w749) -> (w752:string[])
      n347 = Build Array(w752) -> (w750:string[][])
    }
    frame 62250 {
      # "Check"
      n348 = Index Array(array=w757, index=85) -> (element=w759:string)
      n349 = call "Q5 Format.vi"("Data (U16 or U32)"=w761) -> ("Q5 Format Data"=w755:string)  [unwired: 10 in]
      n350 = Build Array(w759, w755) -> (w758:string[])
      n351 = Build Array(w758) -> (w756:string[][])
    }
    frame 62253 {
      # "Partial Coast Time (0xF32D)"
      # "Check"
      n352 = Index Array(array=w764, index=81) -> (element=w766:string)
      n353 = Build Array(w766, w762) -> (w765:string[])
      n354 = Build Array(w765) -> (w763:string[][])
    }
    frame 62254 {
      # "Ramp Line Voltage (0xF32E)"
      # "Check"
      n355 = Index Array(array=w771, index=82) -> (element=w773:string)
      n356 = call "Q5 Format.vi"("Data (U16 or U32)"=w769) -> ("Q5 Format Data"=w768:string)  [unwired: 10 in]
      n357 = Build Array(w773, w768) -> (w772:string[])
      n358 = Build Array(w772) -> (w770:string[][])
    }
    frame 61440 {
      # "Personality (0xF000)"
      n359 = Index Array(array=w777, index=83) -> (element=w779:string)
      n360 = Build Array(w779, w775) -> (w778:string[])
      n361 = Build Array(w778) -> (w776:string[][])
    }
    frame 61463 {
      # "Reset Source (0xF017)"
      # "Check"
      # "Line Number"
      # "File Name CRC"
      n362 = String Subset(string=w791, offset (0)=0, length (rest)=5 ("length (rest)")) -> (substring=w787:string)
      n363 = String Subset(string=w791, offset (0)=6, length (rest)=2 ("length (rest)")) -> (substring=w796:string)
      n364 = String Subset(string=w791, offset (0)=9, length (rest)=2 ("length (rest)")) -> (substring=w797:string)
      n365 = Concatenate Strings(w796, w797) -> (w798:string)
      n366 = Index Array(array=w782, index=84) -> (element=w785:string)
      n367 = Hexadecimal String To Number(string=w798) -> (number=w789:u32)  [unwired: 2 in, 1 out]
      n368 = Number To Decimal String(number=w789) -> (decimal integer string=w788:string)  [unwired: 1 in]
      n369 = call <vilib>:"Space Constant.vi"() -> ("String"=w790:string)
      n370 = Concatenate Strings(w787, w790, w788) -> (w783:string)
      n371 = Build Array(w785, w783) -> (w784:string[])
      n372 = Build Array(w784) -> (w781:string[][])
    }
  }
  "Array" <- w4
